vi "Write slitPosition.vi"(8 "error in (no error)":errorcluster, 10 "slitPosition":T1, 11 "ChangeSlitWidth in":refnum<class "ChangeSlitWidth.lvclass">) -> (0 "error out":errorcluster, 3 "ChangeSlitWidth out":refnum<class "ChangeSlitWidth.lvclass">)   [LabVIEW 2016, in "ChangeSlitWidth.lvclass"]
uses:
  ChangeSlitWidth.lvclass
  Typedefs/slit.ctl
  Typedefs/SlitType.ctl
  Typedefs/slitWidth.ctl
  ChangeSlitWidth.lvclass/ChangeSlitWidth.ctl
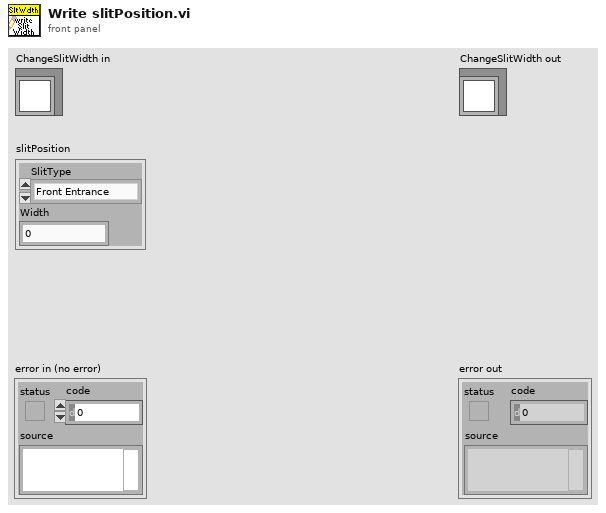
[diagram p1: front panel]
types:
  T1 = typedef "slit.ctl" = cluster{"SlitType":T2, "Width":T3}
  T2 = typedef "SlitType.ctl" = enum16{"Front Entrance", "Side Entrance", "Front Exit", "Side Exit", "First Intermediate", "Second Intermediate"}
  T3 = typedef "slitWidth.ctl" = dbl
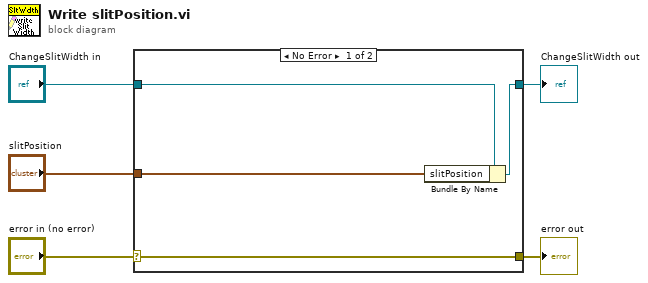
[diagram p0: block diagram]
diagram:
  n1 = case shown="No Error" "error in (no error)" {
    selector: "error in (no error)" -> [w9 w10]
    tunnel: [w9 w10] -> w4
    tunnel: [w7 w11] -> w2
    tunnel: "ChangeSlitWidth in" -> [w8 w11]
    tunnel: "slitPosition" -> [w6 _]
    frame No Error {
      n2 = Bundle By Name(cluster=w8, "slitPosition"=w6) -> (w7:refnum<class "ChangeSlitWidth.lvclass">)
    }
    frame Error {
    }
  }
  "error out" <- w4
  "ChangeSlitWidth out" <- w2
